vi "Gas_Utility.vi"(9 "increment":dbl=0.05 format="%#_13g", 11 "GAS":bool) -> (3 "coerced":dbl)   [LabVIEW 2015]
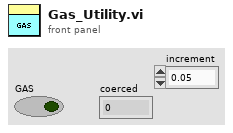
[diagram p1: front panel]
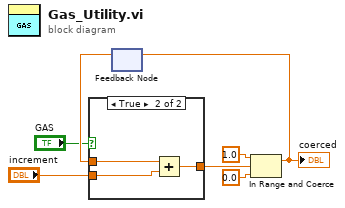
[diagram p0: block diagram]
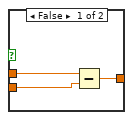
[diagram p2: hidden frame]
diagram:
  n1 = feedback #1() -> (w4:dbl)  [unwired: 1 in]
  n2 = case shown="True" "GAS" {
    tunnel: [w9 w13] -> w3
    tunnel: w4 -> [w10 w12]
    tunnel: "increment" -> [w8 w11]
    frame False {
      n3 = Subtract(x=w10, y=w8) -> (x-y=w9:dbl)
    }
    frame True {
      n4 = Add(x=w12, y=w11) -> (x+y=w13:dbl)
    }
  }
  n5 = In Range and Coerce(upper limit=1.0, x=w3, lower limit=0.0) -> (coerced(x)=w1:dbl)  [unwired: 1 out]
  "coerced" <- w1
  n6 = feedback-in #1(w1) -> ()
